vi "find readout time.vi"(8 "error in (no error)":errorcluster, 11 "Simulated_CCD_Camera in":refnum<class "Simulated Camera.lvclass">) -> (0 "error out":errorcluster, 3 "Simulated_CCD_Camera out":refnum<class "Simulated Camera.lvclass">)   [LabVIEW 2018, in "Simulated Camera.lvclass"]
doc: "Find the readout time as a function of the operation mode of the CCD.\n\nThis value is used to determine the minimum exposure time allowed by ACS, that is the readout time plus 10 % of this value. This procedure is related to the functioning of the frame transfer mode of the CCD and it prevents the misuse of the exposure time."
uses:
  Simulated Camera.lvclass
  Simulated Camera.lvclass/Simulated Camera.ctl
  <vilib>/Utility/file.llb/Read Delimited Spreadsheet (DBL).vi
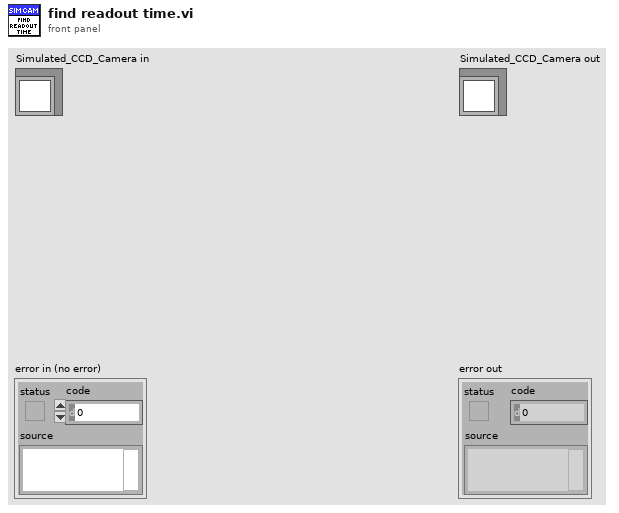
[diagram p1: front panel]
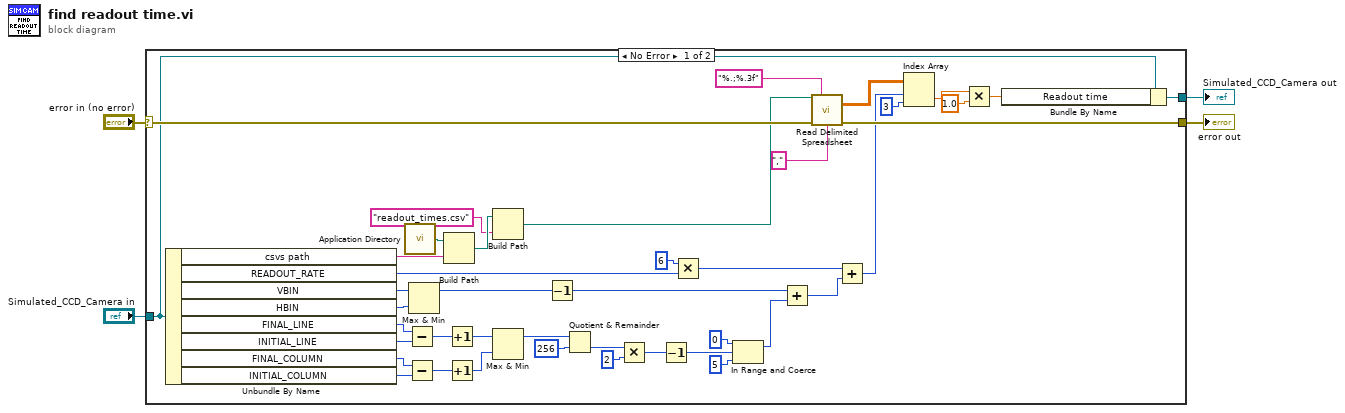
[diagram p0: block diagram]
diagram:
  n1 = case shown="No Error" "error in (no error)" {
    selector: "error in (no error)" -> [w46 w48]
    tunnel: [w45 w48] -> w3
    tunnel: [w11 w47] -> w1
    tunnel: "Simulated_CCD_Camera in" -> [w12 w47]
    frame No Error {
      n2 = Unbundle By Name(w12) -> ("csvs path"=w5:string, "READOUT_RATE"=w28:u16, "VBIN"=w32:u16, "HBIN"=w31:u16, "FINAL_LINE"=w40:u16, "INITIAL_LINE"=w39:u16, "FINAL_COLUMN"=w38:u16, "INITIAL_COLUMN"=w37:u16)
      n3 = call <vilib>:"Application Directory.vi"() -> ("Application Directory"=w43:path)
      n4 = Subtract(x=w40, y=w39) -> (x-y=w42:u16)
      n5 = Subtract(x=w38, y=w37) -> (x-y=w41:u16)
      n6 = Max & Min(x=w32, y=w31) -> (max(x,y)=w30:u16)  [unwired: 1 out]
      n7 = Build Path(base path=w43, name or relative path=w5) -> (appended path=w9:path)
      n8 = Increment(x=w42) -> (x+1=w36:u16)
      n9 = Increment(x=w41) -> (x+1=w35:u16)
      n10 = Build Path(base path=w9, name or relative path="readout_times.csv") -> (appended path=w8:path)
      n11 = Max & Min(x=w36, y=w35) -> (max(x,y)=w33:u16)  [unwired: 1 out]
      n12 = Decrement(x=w30) -> (x-1=w29:u16)
      n13 = Quotient & Remainder(x=w33, y=u16 256) -> (floor(x/y)=w19:u16)  [unwired: 1 out]
      n14 = Multiply(x=w19, y=u16 2 ("x")) -> (x*y=w20:u16)
      n15 = Decrement(x=w20) -> (x-1=w18:u16)
      n16 = Multiply(x=u16 6, y=w28) -> (x*y=w25:u16)
      n17 = In Range and Coerce(upper limit=u16 0, x=w18, lower limit=u16 5 ("upper limit")) -> (coerced(x)=w15:u16)  [unwired: 1 out]
      n18 = Add(x=w29, y=w15) -> (x+y=w26:u16)
      n19 = call-poly <vilib>:"Read Delimited Spreadsheet.vi"("file path (dialog if empty)"=w8, "format (%.3f)"="%.;%.3f", "error in (no error)"=w46, "delimiter (\\t)"="," ("delimiter (\\t)")) -> ("all rows"=w23:dbl[][], "error out"=w45:errorcluster)  [unwired: 6 in, 4 out]
      n20 = Add(x=w25, y=w26) -> (x+y=w24:u16)
      n21 = Index Array(array=w23, index (row)=w24, index (col)=3 ("disabled index (col)")) -> (element=w14:dbl)
      n22 = Multiply(x=w14, y=1.0) -> (x*y=w10:dbl)
      n23 = Bundle By Name(cluster=w12, "Readout time"=w10) -> (w11:refnum<class "Simulated Camera.lvclass">)
    }
    frame Error {
    }
  }
  "error out" <- w3
  "Simulated_CCD_Camera out" <- w1
